vi "SMO.InstrumentDriver.SetConfiguration.vi"(8 "error in (no error)":errorcluster, 10 "Configuration":variant, 11 "SMO.Instrument":refnum<class "SMO.InstrumentDriver.lvclass">) -> (0 "error out":errorcluster, 3 "SMO.Instrument out":refnum<class "SMO.InstrumentDriver.lvclass">)   [LabVIEW 2013, in "SMO.InstrumentDriver.lvclass"]
doc: "---------------------------------------------------------------\nJKI State Machine Objects™\nhttp://jki.net/state-machine-objects/\nCopyright (C) 2005-2015, JKI <info@jki.net>\nALL RIGHTS RESERVEDJKI State Machine Objects (SMO) 1.0.0.5\nJKI - JKI\nCopyright (c) 2016, JKI"
uses:
  SMO.InstrumentDriver.lvclass
  Typedefs/Configuration--Cluster.ctl
  SMO.InstrumentDriver.lvclass/SMO.InstrumentDriver.ctl
panel:
  # "For instructions on how to use the JKI State Machine Objects, examples and video tutorials, visit:\nhttp://jki.net/state-machine-objects/\n\nJKI State Machine Objects™\nhttp://jki.net/state-machine-objects/\nCopyright (C) 2005-2015, JKI <info@jki.net>\nALL RIGHTS RESERVED"
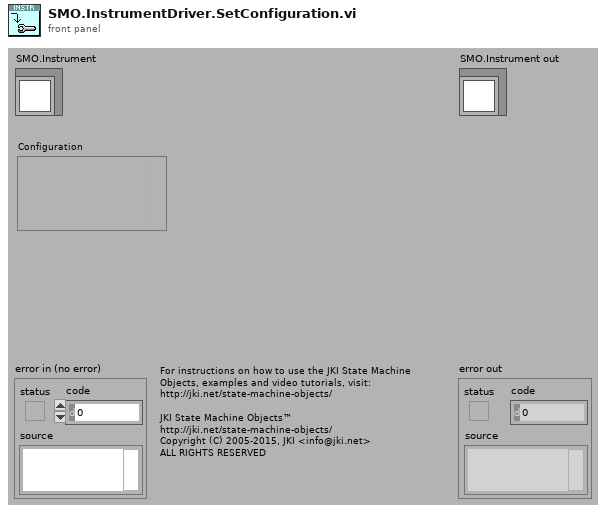
[diagram p1: front panel]
types:
  T1 = typedef "SMO.InstrumentDriver.lvclass/Configuration--Cluster.ctl" = cluster{"Polling Rate (ms)":i32}
  T2 = typedef "SMO.InstrumentDriver.lvclass/PrivateData--Ref.ctl" = refnum<data-value>
  T3 = typedef "SMO.InstrumentDriver.lvclass/PrivateData--Cluster.ctl" = cluster{"Public Events":T4, "Configuration":T1}
  T4 = typedef "SMO.InstrumentDriver.lvclass/PublicEvents--Cluster.ctl" = cluster{"Value Changed":refnum<user-event>}
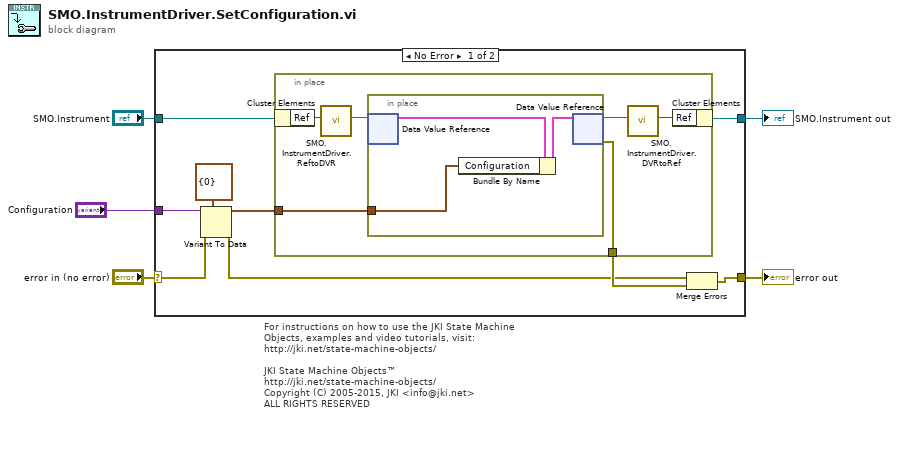
[diagram p0: block diagram]
diagram:
  # "For instructions on how to use the JKI State Machine Objects, examples and video tutorials, visit:\nhttp://jki.net/state-machine-objects/\n\nJKI State Machine Objects™\nhttp://jki.net/state-machine-objects/\nCopyright (C) 2005-2015, JKI <info@jki.net>\nALL RIGHTS RESERVED"
  n1 = case shown="No Error" "error in (no error)" {
    selector: "error in (no error)" -> [w7 w24]
    tunnel: "SMO.Instrument" -> [w11 w25]
    tunnel: [w12 w24] -> w4
    tunnel: [w14 w25] -> w3
    tunnel: "Configuration" -> [w10 _]
    frame No Error {
      n2 = Variant To Data(error in=w7, type=T1 {"Polling Rate (ms)"=0} ("Configuration"), Variant=w10) -> (data=w8:T1, error out=w6:errorcluster)
      n3 = in-place {
        in-place-border: [w20] -> w13
        in-place-border: w8 -> [w15]
        n4 = in-place-cluster #1(w11) -> ("Ref"=w19:u32)
        n5 = call "SMO.InstrumentDriver.ReftoDVR.vi"("Ref"=w19) -> ("Ref"=w18:T2)  [unwired: 10 in]
        n6 = in-place {
          in-place-border: w15 -> [w21]
          n7 = in-place-dvr #2(w18) -> (w23:T3)  [unwired: 1 out]
          n8 = Bundle By Name(cluster=w23, "Configuration"=w21) -> (w22:T3)
          n9 = in-place-dvr #2(w22) -> (w17:T2, w20:errorcluster)
        }
        n10 = call "SMO.InstrumentDriver.DVRtoRef.vi"("Ref"=w17) -> ("Ref"=w16:u32)  [unwired: 10 in]
        n11 = in-place-cluster #1("Ref"=w16) -> (w14:refnum<class "SMO.InstrumentDriver.lvclass">)
      }
      n12 = Merge Errors(w6, w13) -> (w12:errorcluster)
    }
    frame Error {
    }
  }
  "error out" <- w4
  "SMO.Instrument out" <- w3
